vi "Do Write.vi"(8 "error in (no error)":errorcluster, 10 "Interface":refnum<class "Interface.lvclass">, 11 "Section 2a in":refnum<class "Section 2a.lvclass">) -> (0 "error out":errorcluster, 3 "Section 2a out":refnum<class "Section 2a.lvclass">, 4 "All Keys Found?":bool)   [LabVIEW 2012, in "LVOOP Introduction.lvlib" / "Section 2a.lvclass"]
doc: "Write keys/value pairs to Interface.\n\nOverwriting dynamic dispatch VI."
uses:
  Section 2a.lvclass
  Configuration/Classes/Interface/Interface.lvclass
  Section 2/Section 2.lvclass
  Section 2a.lvclass/Section 2a.ctl
  Configuration/Classes/Section/Section.lvclass
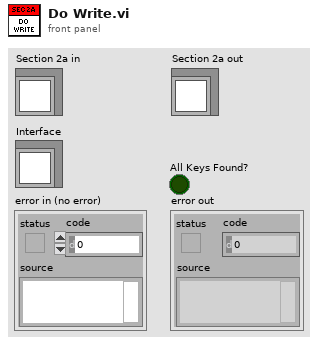
[diagram p1: front panel]
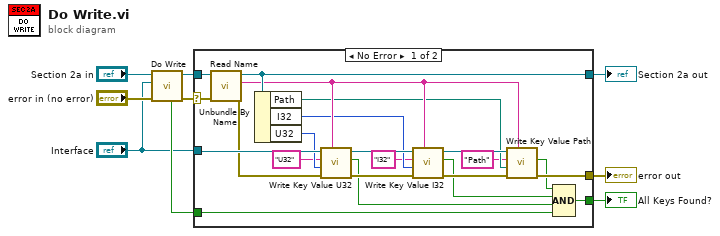
[diagram p0: block diagram]
diagram:
  n1 = call-parent "Do Write.vi"("error in (no error)"="error in (no error)", "Interface"="Interface", "Section 2 in"="Section 2a in") -> ("error out"=w3:errorcluster, "Section 2 out"=w4:refnum<class "Section 2a.lvclass">, "All Keys Found?"=w2:bool)  [unwired: 6 in]
  n2 = case shown="No Error" w3 {
    selector: w3 -> [w11 w32]
    tunnel: w4 -> [w12 w33]
    tunnel: [w31 w33] -> w9
    tunnel: "Interface" -> [w30 _]
    tunnel: [w19 w32] -> w8
    tunnel: [w13 _] -> w7
    tunnel: w2 -> [w10 _]
    frame No Error {
      n3 = call "Read Name.vi"("error in (no error)"=w11, "Section in"=w12) -> ("error out"=w21:errorcluster, "Name"=w27:string, "Section out"=w31:refnum<class "Section 2a.lvclass">)  [unwired: 7 in]
      n4 = Unbundle By Name(w31) -> ("Path"=w24:path, "I32"=w25:i32, "U32"=w26:u32)
      n5 = call-dynamic "Write Key Value U32.vi"("Section Name"=w27, "error in (no error)"=w21, "Value"=w26, "Key Name"="U32", "Interface in"=w30) -> ("error out"=w22:errorcluster, "found"=w14:bool, "Interface out"=w29:refnum<class "Interface.lvclass">)  [unwired: 4 in]
      n6 = call-dynamic "Write Key Value I32.vi"("Section Name"=w27, "error in (no error)"=w22, "Value"=w25, "Key Name"="I32", "Interface in"=w29) -> ("error out"=w20:errorcluster, "found"=w15:bool, "Interface out"=w28:refnum<class "Interface.lvclass">)  [unwired: 4 in]
      n7 = call-dynamic "Write Key Value Path.vi"("Section Name"=w27, "error in (no error)"=w20, "Value"=w24, "Key Name"="Path", "Interface in"=w28) -> ("error out"=w19:errorcluster, "found"=w16:bool)  [unwired: 4 in, 1 out]
      n8 = Compound Arithmetic op=AND(w16, w15, w14, w10) -> (w13:bool)
    }
    frame Error {
    }
  }
  "error out" <- w8
  "Section 2a out" <- w9
  "All Keys Found?" <- w7
